vi "Select DMM Current Range.vi"(8 "error in (no error)":errorcluster, 11 "Max":dbl) -> (0 "error out":errorcluster, 2 "1A/10A?":bool, 3 "DMM current range":dbl)   [LabVIEW 2018]
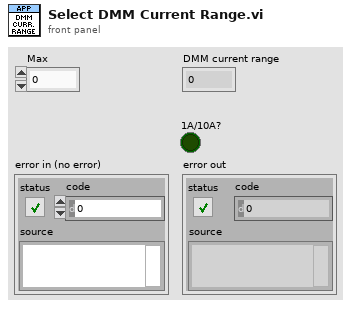
[diagram p1: front panel]
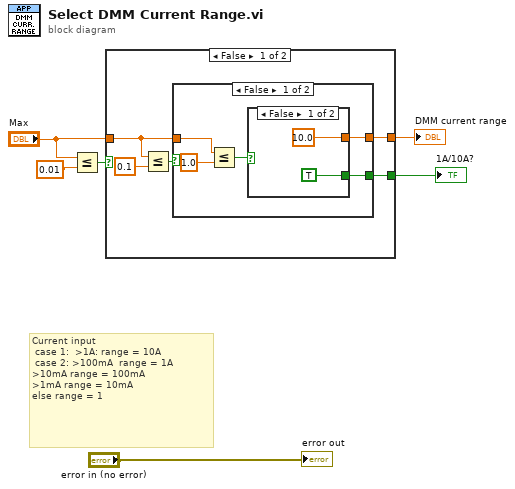
[diagram p0: block diagram]
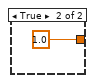
[diagram p2: hidden frame]
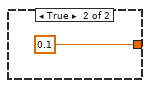
[diagram p3: hidden frame]
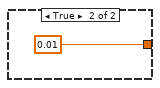
[diagram p4: hidden frame]
diagram:
  # "Current input\n case 1:  >1A: range = 10A\n case 2: >100mA  range = 1A\n>10mA range = 100mA\n>1mA range = 10mA\nelse range = 1"
  n1 = Less Or Equal?(x="Max", y=0.01) -> (x <= y?=w4:bool)
  n2 = case shown="False" w4 {
    tunnel: "Max" -> [w8 _]
    tunnel: [w9 0.01] -> w2
    tunnel: [w7 _] -> w1
    frame False {
      n3 = Less Or Equal?(x=w8, y=0.1) -> (x <= y?=w11:bool)
      n4 = case shown="False" w11 {
        tunnel: [w13 0.1] -> w9
        tunnel: w8 -> [w16 _]
        tunnel: [w12 _] -> w7
        frame False {
          n5 = Less Or Equal?(x=w16, y=1.0) -> (x <= y?=w14:bool)
          n6 = case shown="False" w14 {
            tunnel: [10.0 1.0] -> w13
            tunnel: [TRUE _] -> w12
            frame False {
            }
            frame True {
            }
          }
        }
        frame True {
        }
      }
    }
    frame True {
    }
  }
  "1A/10A?" <- w1
  "DMM current range" <- w2
  "error out" <- "error in (no error)"
